vi "E441X_PM_Configure_Limits.vi"(0 "VISA session":refnum<visa-resource-name>, 1 "Measurement (1)":i32=1, 5 "State (T: On)":bool=TRUE, 7 "Auto Clear (1: On)":i32(ring)=1 items=["Off", "On", "ONCE"], 11 "error in (no error)":errorcluster {"code" format="%.0x"}, 12 "Lower Limit (-90.00E+0)":dbl=-90.0 format="%^.2e", 13 "Upper Limit (90.00E+0)":dbl=90.0 format="%^.2e") -> (4 "dup VISA session":refnum<visa-resource-name>, 15 "error out":errorcluster {"code" format="%.0x"})   [LabVIEW 2015]
doc: "This VI configures parameters of limits. This limits are used for TTL logic level output on the rear panel TTL Input/Output connector.\n\nNotes:\n(1) For limits failure checking see VI Get Limits Failure."
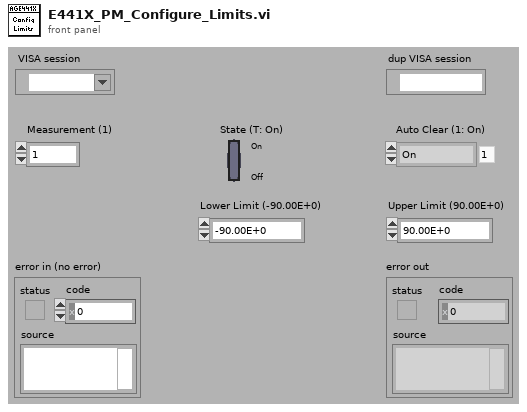
[diagram p1: front panel]
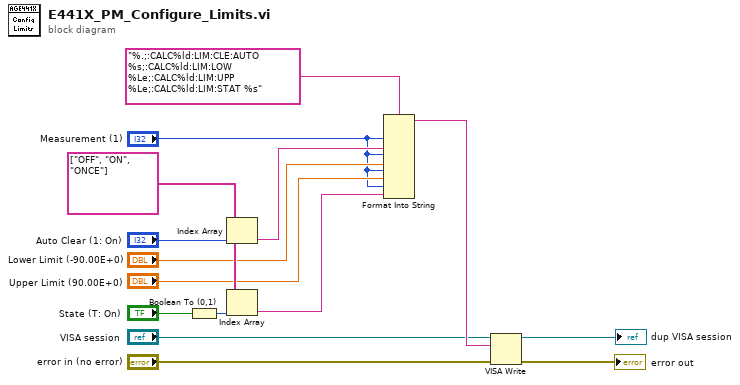
[diagram p0: block diagram]
diagram:
  w14 = string[] ["OFF", "ON", "ONCE"]
  n1 = Boolean To (0,1)(Boolean="State (T: On)") -> (0, 1=w8:i16)
  n2 = Index Array(array=w14, index="Auto Clear (1: On)") -> (element=w12:string)
  n3 = Index Array(array=w14, index=w8) -> (element=w6:string)
  n4 = Format Into String(format string="%.;:CALC%ld:LIM:CLE:AUTO %s;:CALC%ld:LIM:LOW %Le;:CALC%ld:LIM:UPP %Le;:CALC%ld:LIM:STAT %s", "Measurement (1)", w12, "Measurement (1)", "Lower Limit (-90.00E+0)", "Measurement (1)", "Upper Limit (90.00E+0)", "Measurement (1)", w6) -> (resulting string=w5:string)  [unwired: 2 in, 1 out]
  n5 = VISA Write(VISA resource name="VISA session", write buffer=w5, error in (no error)="error in (no error)") -> (VISA resource name out=→"dup VISA session":refnum<visa-resource-name>, error out=→"error out":errorcluster)  [unwired: 1 out]
